vi "initialize Session Data.vi"(0 "OBJ - Session in":refnum<class "File Session.lvclass">, 11 "error in":errorcluster) -> (4 "OBJ - Session out":refnum<class "File Session.lvclass">, 15 "error out":errorcluster)   [LabVIEW 2019, in "File Session.lvclass"]
doc: "OVERRIDE VI\nPlaceholder for decendant sessions to initialize and set their default values"
uses:
  File Session.lvclass
  File Session.lvclass/File Session.ctl
  Accessors/Read Path.vi
  Create (Replace) File.vi
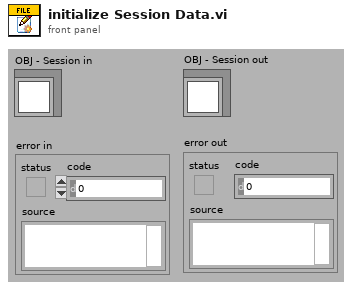
[diagram p1: front panel]
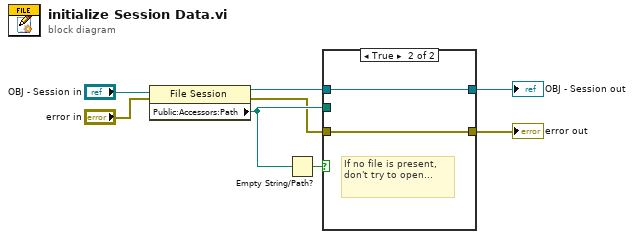
[diagram p0: block diagram]
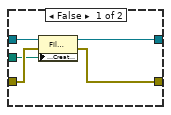
[diagram p2: hidden frame]
diagram:
  n1 = property class="File Session"(reference="OBJ - Session in", error in="error in") -> (reference out=w5:refnum<class "File Session.lvclass">, error out=w3:errorcluster, "Public:Accessors:Path"=w4:path)
  n2 = Empty String/Path?(string/path=w4) -> (empty?=w6:bool)
  n3 = case shown="True" w6 {
    tunnel: w4 -> [w9 _]
    tunnel: w3 -> [w13 w14]
    tunnel: w5 -> [w12 w15]
    tunnel: [w11 w15] -> w2
    tunnel: [w10 w14] -> w1
    frame False {
      n4 = property class="File Session"(reference=w12, error in=w13, "Public:Create (Replace) File"=w9) -> (reference out=w11:refnum<class "File Session.lvclass">, error out=w10:errorcluster)
    }
    frame True {
      # "If no file is present, don't try to open..."
    }
  }
  "error out" <- w1
  "OBJ - Session out" <- w2
